vi "Set Acyclic Buffer ID.vi"(8 "error in":errorcluster, 10 "acyclic buffer ID":string, 11 "acyclic frame trigger in":T1 format="%.0x") -> (0 "error out":errorcluster, 3 "acyclic frame trigger out":T1 format="%.0x")   [LabVIEW 2020, in "Ballard MIL-STD-1553 Scripting.lvlib"]
uses:
  Ballard MIL-STD-1553 Scripting.lvlib
  <vilib>/NI VeriStand/Custom Device API/Custom Device Item Ref.ctl
  Constants.vi
  <vilib>/NI VeriStand/Custom Device API/Set Item Property (String).vi
  <vilib>/NI VeriStand/Custom Device API/Custom Device API.lvlib
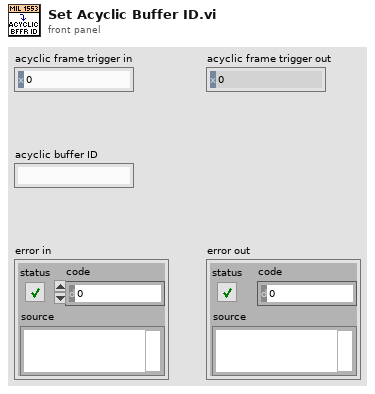
[diagram p1: front panel]
types:
  T1 = typedef "Custom Device API.lvlib/Custom Device Item Ref.ctl" = u64
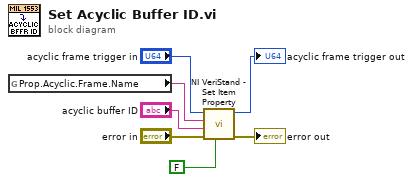
[diagram p0: block diagram]
diagram:
  n1 = global read "Constants.vi" "Prop.Acyclic.Frame.Name"() -> (w7:string)
  n2 = call-poly <vilib>:"NI VeriStand - Set Item Property.vi"("Binary String (T)"=FALSE, "error in (no error)"="error in", "Value"="acyclic buffer ID", "Property Name"=w7, "Item Ref in"="acyclic frame trigger in") -> ("error out"=→"error out":errorcluster, "Item Ref out"=→"acyclic frame trigger out":T1)  [unwired: 4 in, 1 out]
